vi "HW File config.vi"(10 "base path":path) -> (0 "Cancel":bool, 2 "count":string caption="选择文件")   [LabVIEW 2018]
panel:
  in  "取消":bool
  in  "OK":bool
  in  "配置硬件列表":i32(listbox)
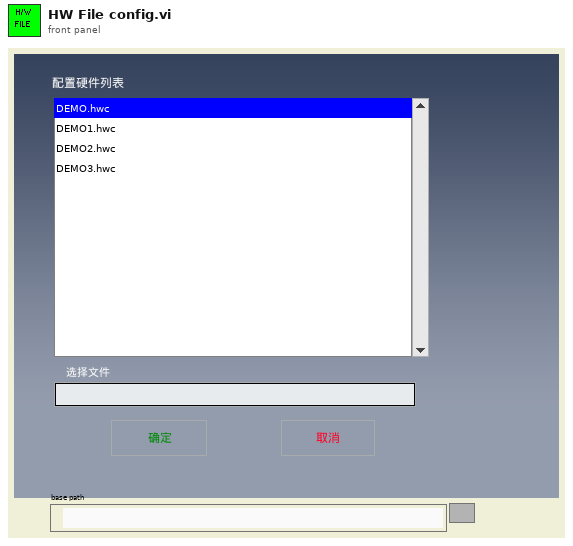
[diagram p1: front panel]
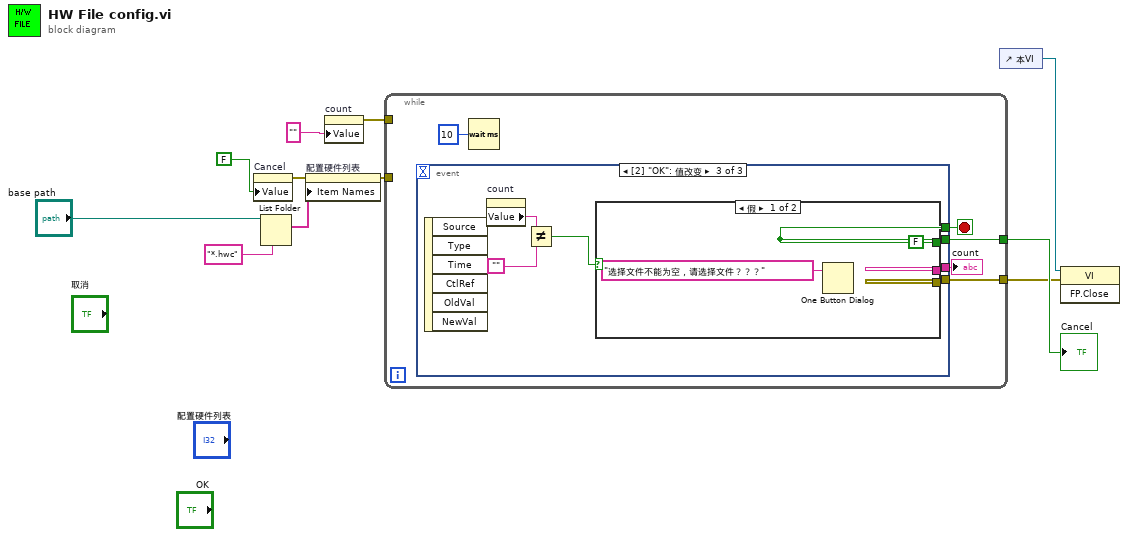
[diagram p0: block diagram]
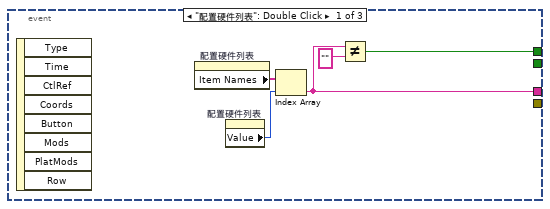
[diagram p2: hidden frame]
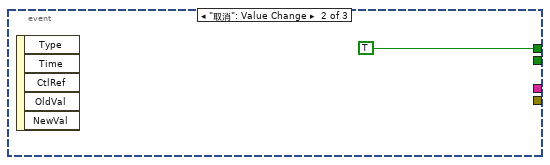
[diagram p3: hidden frame]
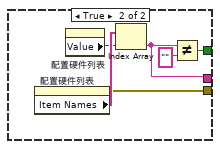
[diagram p4: hidden frame]
diagram:
  n1 = property on="Cancel" class="Bool (严格)"("Value"=FALSE) -> (error out=w4:errorcluster)  [unwired: 2 in, 1 out]
  n2 = List Folder(path="base path", pattern="*.hwc") -> (filenames=w11:string[])  [unwired: 1 in, 4 out]
  n3 = property on="配置硬件列表" class="LstBox (严格)"(error in=w4, "Item Names"=w11) -> (error out=w10:errorcluster)  [unwired: 1 in, 1 out]
  n4 = property on="count" class="Str"("Value"="") -> (error out=w8:errorcluster)  [unwired: 2 in, 1 out]
  n5 = while {
    tunnel: w10 -> [_]
    tunnel: w8 -> [_]
    tunnel: [w14] -> w5
    tunnel: [w12] -> w1
    stop <- w15 stop-if-true
    n6 = event shown="[2] \"OK\": 值改变" {
      selector: _ -> [_ _ _]
      dyn-events: _ -> [_ _ _]
      timeout: _ -> [_ _ _]
      tunnel: [w18 TRUE w27] -> w15
      tunnel: [_ _ w27] -> w14
      tunnel: [w17 _ w28] -> w13
      tunnel: [_ _ w26] -> w12
      event "配置硬件列表": Double Click {
        n7 = event-data() -> ()  [unwired: 9 out]
        n8 = property on="配置硬件列表" class="LstBox (严格)"() -> ("Item Names"=w21:string[])  [unwired: 2 in, 2 out]
        n9 = property on="配置硬件列表" class="LstBox (严格)"() -> ("Value"=w20:i32)  [unwired: 2 in, 2 out]
        n10 = Index Array(array=w21, index=w20) -> (element=w17:string)
        n11 = Not Equal?(x=w17, y="") -> (x != y?=w18:bool)
      }
      event "取消": Value Change {
        n12 = event-data() -> ()  [unwired: 6 out]
      }
      event "OK": Value Change {
        n13 = event-data() -> ()  [unwired: 7 out]
        n14 = property on="count" class="Str"() -> ("Value"=w24:string)  [unwired: 2 in, 2 out]
        n15 = Not Equal?(x=w24, y="") -> (x != y?=w25:bool)
        n16 = case shown="假" w25 {
          tunnel: [_ w33] -> w28
          tunnel: [FALSE w32] -> w27
          tunnel: [_ w31] -> w26
          frame False {
            n17 = One Button Dialog(message="选择文件不能为空，请选择文件？？？" ("消息")) -> ()  [unwired: 1 in, 1 out]
          }
          frame True {
            n18 = property on="配置硬件列表" class="LstBox (严格)"() -> (error out=w31:errorcluster, "Item Names"=w36:string[])  [unwired: 2 in, 1 out]
            n19 = property on="配置硬件列表" class="LstBox (严格)"() -> ("Value"=w35:i32)  [unwired: 2 in, 2 out]
            n20 = Index Array(array=w36, index=w35) -> (element=w33:string)
            n21 = Not Equal?(x=w33, y="") -> (x != y?=w32:bool)
          }
        }
      }
    }
    "count" <- w13
    n22 = Wait (ms)(milliseconds to wait=u32 10) -> ()  [unwired: 1 out]
  }
  "Cancel" <- w5
  n23 = control-ref of="本VI"() -> (w2:refnum<vi>)
  n24 = invoke class="VI" method="FP.Close"(reference=w2, error in=w1) -> ()  [unwired: 1 in, 3 out]
